vi "Car_Speed_R563X.vi"(10 "精度":dbl=0.0625, 11 "车速":u16) -> (3 "报文":T1 {"[7]" format="%02x"; "[6]" format="%02x"; "[5]" format="%02x"; "[4]" format="%02x"; "[3]" format="%02x"; "[2]" format="%02x"; "[1]" format="%02x"; "[0]" format="%02x"})   [LabVIEW 2020]
uses:
  Global_Variable/Global.vi
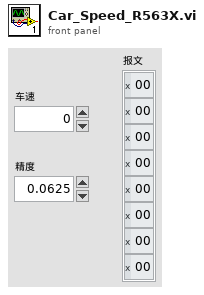
[diagram p1: front panel]
types:
  T1 = cluster{"[0]":u8, "[1]":u8, "[2]":u8, "[3]":u8, "[4]":u8, "[5]":u8, "[6]":u8, "[7]":u8}
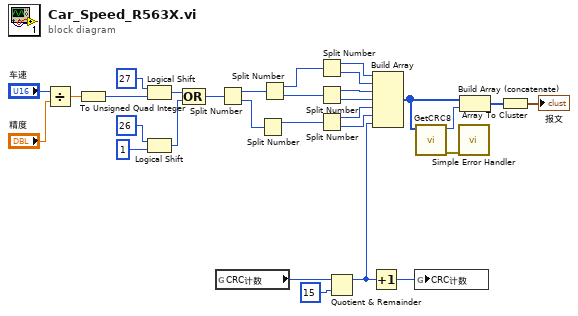
[diagram p0: block diagram]
diagram:
  n1 = Divide(x="车速", y="精度") -> (x/y=w27:dbl)
  n2 = To Unsigned Quad Integer(1:w27) -> (0:w5:u64)
  n3 = Logical Shift(y=i16 27, x=w5) -> (x << y=w17:u64)
  n4 = Logical Shift(y=i16 26, x=u64 1) -> (x << y=w19:u64)
  n5 = Compound Arithmetic op=OR ("复合运算")(w17, w19) -> (w16:u64)
  n6 = global read "Global.vi" "CRC计数"() -> (w2:u8)
  n7 = Split Number(x=w16) -> (hi(x)=w25:u32, lo(x)=w24:u32)
  n8 = Split Number(x=w24) -> (hi(x)=w21:u16)  [unwired: 1 out]
  n9 = Split Number(x=w25) -> (hi(x)=w23:u16, lo(x)=w22:u16)
  n10 = Split Number(x=w23) -> (hi(x)=w15:u8, lo(x)=w14:u8)
  n11 = Split Number(x=w22) -> (hi(x)=w13:u8, lo(x)=w12:u8)
  n12 = Split Number(x=w21) -> (hi(x)=w11:u8, lo(x)=w10:u8)
  n13 = Quotient & Remainder(x=w2, y=u8 15) -> (x-y*floor(x/y)=w3:u8)  [unwired: 1 out]
  n14 = Increment(x=w3) -> (x+1=w1:u8)
  n15 = Build Array(w15, w14, w13, w12, w11, w10, w3) -> (w9:u8[])
  n16 = global write "Global.vi" "CRC计数"(w1) -> ()
  n17 = call "GetCRC8.vi"("xData"=w9) -> ("错误输出"=w6:errorcluster, "CRC8"=w8:u8)  [unwired: 9 in]
  n18 = call <vilib>:"Simple Error Handler.vi"("error in (no error)"=w6) -> ()  [unwired: 4 in, 5 out]
  n19 = Build Array (concatenate)(w9, w8) -> (w7:u8[])
  n20 = Array To Cluster(array=w7) -> (cluster=→"报文":T1)
